vi "WriteToServer.vi"(0 "TCP in":refnum<k5>, 7 "Command":string, 11 "error in":errorcluster, 12 "Timeout(1000ms)":i32=1000) -> (4 "TCP out":refnum<k5>, 6 "ReplyData":T1, 10 "Reply Type":T2, 15 "error out":errorcluster)   [LabVIEW 2020, in "Redis.lvclass"]
uses:
  Redis.lvclass
  ReplyDataTypeEnum.ctl
  ReplyDataType.ctl
  Redis.lvclass/Redis.ctl
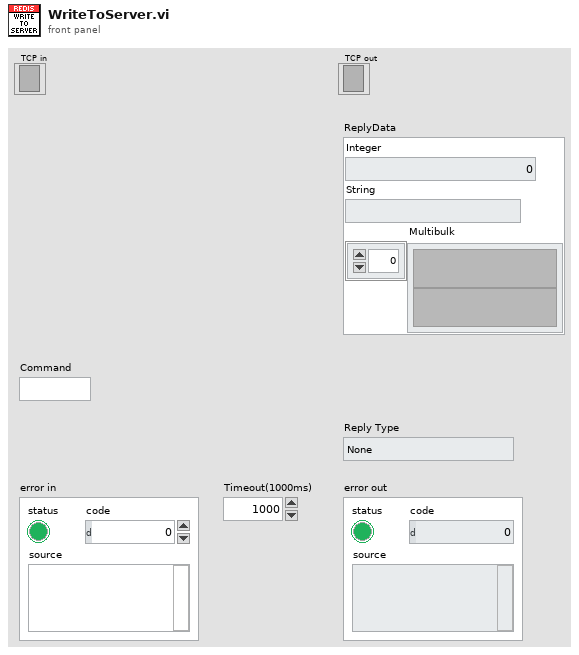
[diagram p1: front panel]
types:
  T1 = typedef "Redis.lvclass/ReplyDataType.ctl" = cluster{"Integer":i64, "String":string, "Multibulk":variant[]}
  T2 = typedef "Redis.lvclass/ReplyDataTypeEnum.ctl" = enum16{"None", "Error", "Status", "Nil", "Integer", "String", "Multibulk"}
  T3 = enum16{"Standard", "Buffered", "CRLF", "Immediate"}
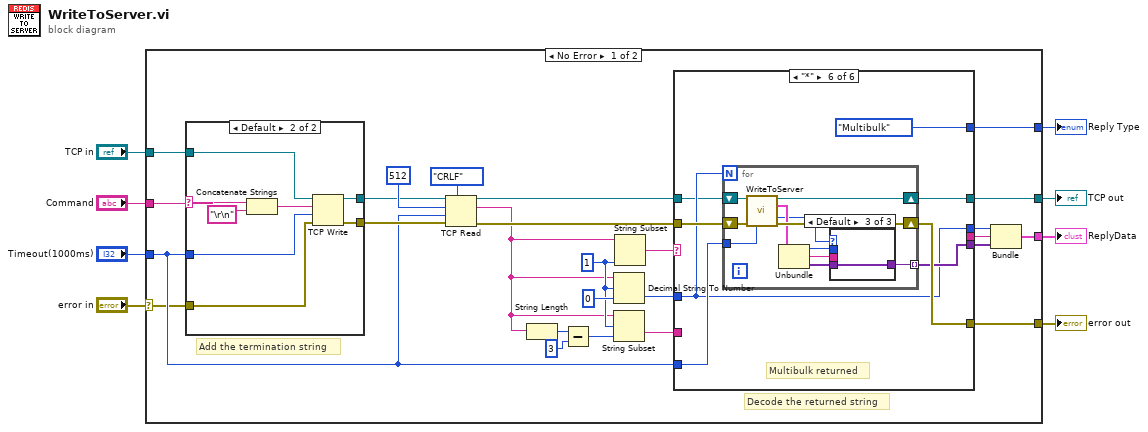
[diagram p0: block diagram]
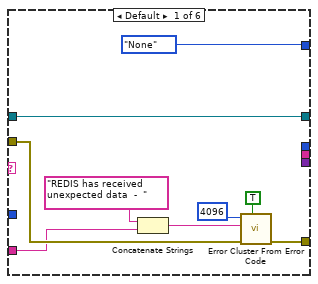
[diagram p3: hidden frame]
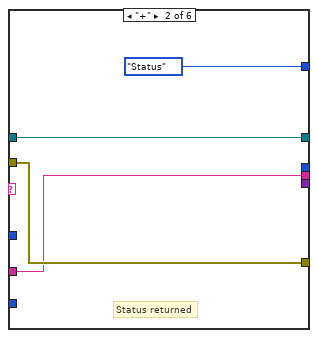
[diagram p4: hidden frame]
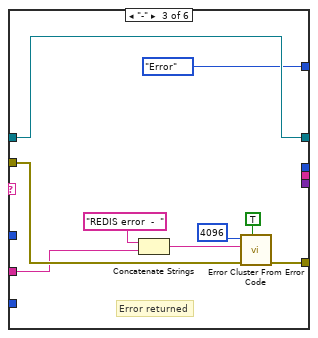
[diagram p5: hidden frame]
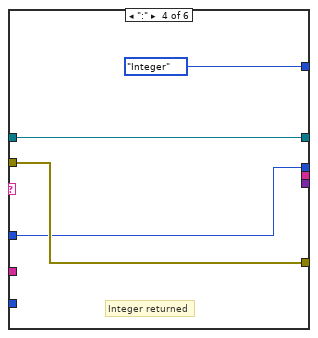
[diagram p6: hidden frame]
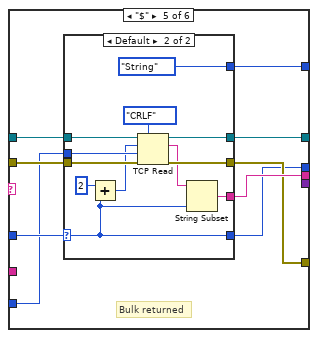
[diagram p7: hidden frame]
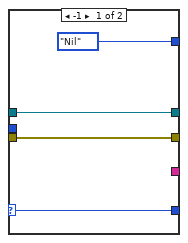
[diagram p8: hidden frame]
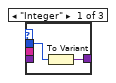
[diagram p9: hidden frame]
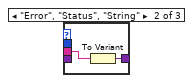
[diagram p10: hidden frame]
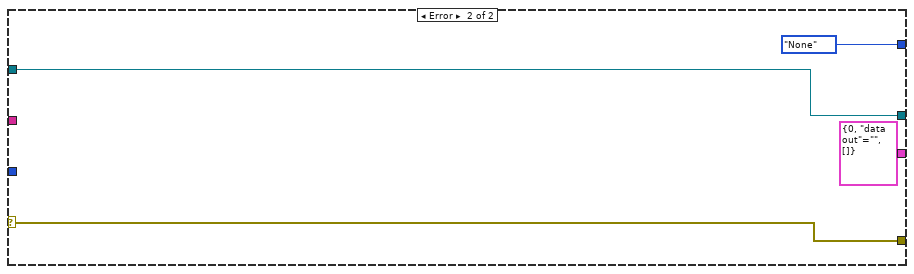
[diagram p11: hidden frame]
diagram:
  n1 = case shown="No Error" "error in" {
    selector: "error in" -> [w9 w122]
    tunnel: [w29 w122] -> w3
    tunnel: [w28 ReplyDataTypeEnum."None" ("Reply Type")] -> w6
    tunnel: "Timeout(1000ms)" -> [w17 _]
    tunnel: "TCP in" -> [w16 w123]
    tunnel: "Command" -> [w15 _]
    tunnel: [w13 cluster{i64, "data out":string, variant[]} {0, "data out"="", []}] -> w1
    tunnel: [w11 w123] -> w7
    frame No Error {
      w24 = 1 ("length (rest)")
      # "Decode the returned string"
      # "Add the termination string"
      n2 = case shown="Default" w15 {
        selector: w15 -> [_ w37]
        tunnel: [w36 w44] -> w12
        tunnel: [w35 w43] -> w18
        tunnel: w9 -> [w35 w42]
        tunnel: w17 -> [_ w41]
        tunnel: w16 -> [w36 w40]
        frame "" {
        }
        frame Default {
          n3 = Concatenate Strings(w37, "\r\n" ("data in")) -> (w39:string)
          n4 = TCP Write(connection ID=w40, data in=w39, error in (no error)=w42, 9:w41) -> (connection ID out=w44:refnum<k5>, error out=w43:errorcluster)  [unwired: 1 out]
        }
      }
      n5 = TCP Read(connection ID=w12, bytes to read=512, error in (no error)=w18, 7:T3."CRLF" ("mode (standard)"), 9:w17) -> (connection ID out=w10:refnum<k5>, data out=w19:string, error out=w30:errorcluster)
      n6 = String Length(string=w19) -> (length=w23:i32)
      n7 = Subtract(x=w23, y=3) -> (x-y=w21:i32)
      n8 = Decimal String To Number(string=w19, offset=w24, default (0L)=i64 0 ("default (0 I32)")) -> (number=w34:i64)  [unwired: 1 out]
      n9 = String Subset(string=w19, offset (0)=w24, length (rest)=w21) -> (substring=w20:string)
      n10 = String Subset(string=w19, length (rest)=w24) -> (substring=w25:string)  [unwired: 1 in]
      n11 = case shown="\"*\"" w25 {
        tunnel: w20 -> [w48 w56 w61 _ _ _]
        tunnel: [_ w56 _ _ w78 _] -> w26
        tunnel: w10 -> [w46 w55 w59 w68 w72 w97]
        tunnel: w34 -> [_ _ _ w69 w79 w99]
        tunnel: [_ _ _ w69 w73 w99] -> w27
        tunnel: [ReplyDataTypeEnum."None" ("Reply Type") ReplyDataTypeEnum."Status" ("Reply Type") ReplyDataTypeEnum."Error" ("Reply Type") ReplyDataTypeEnum."Integer" ("Reply Type") w77 ReplyDataTypeEnum."Multibulk" ("Reply Type")] -> w28
        tunnel: w30 -> [w49 w57 w62 w70 w76 w103]
        tunnel: [w53 w57 w66 w70 w74 w102] -> w29
        tunnel: w17 -> [_ _ _ _ w75 w100]
        tunnel: [_ _ _ _ _ w101] -> w14
        tunnel: [w46 w55 w59 w68 w71 w98] -> w11
        frame Default {
          n12 = Concatenate Strings("REDIS has received unexpected data  -  " ("string"), w48) -> (w51:string)
          n13 = call <vilib>:"Error Cluster From Error Code.vi"("show call chain? (False)"=TRUE, "error in (no error)"=w49, "error message (\"\")"=w51, "error code (0)"=4096) -> ("error out"=w53:errorcluster)  [unwired: 5 in]
        }
        frame "+" {
          # "Status returned"
        }
        frame "-" {
          # "Error returned"
          n14 = Concatenate Strings("REDIS error  -  " ("string"), w61) -> (w64:string)
          n15 = call <vilib>:"Error Cluster From Error Code.vi"("show call chain? (False)"=TRUE, "error in (no error)"=w62, "error message (\"\")"=w64, "error code (0)"=4096) -> ("error out"=w66:errorcluster)  [unwired: 5 in]
        }
        frame ":" {
          # "Integer returned"
        }
        frame "$" {
          # "Bulk returned"
          n16 = case shown="Default" w79 {
            selector: w79 -> [w83 w85]
            tunnel: [_ w87] -> w78
            tunnel: [ReplyDataTypeEnum."Nil" ("Reply Type") ReplyDataTypeEnum."String" ("Reply Type")] -> w77
            tunnel: [w83 w85] -> w73
            tunnel: w76 -> [w82 w94]
            tunnel: w75 -> [_ w93]
            tunnel: [w82 w92] -> w74
            tunnel: w72 -> [w81 w91]
            tunnel: [w81 w86] -> w71
            frame -1 {
            }
            frame Default {
              n17 = Add(x=i64 2, y=w85) -> (x+y=w90:i64)
              n18 = TCP Read(connection ID=w91, bytes to read=w90, error in (no error)=w94, 7:T3."CRLF" ("mode (standard)"), 9:w93) -> (connection ID out=w86:refnum<k5>, data out=w88:string, error out=w92:errorcluster)
              n19 = String Subset(string=w88, length (rest)=w85) -> (substring=w87:string)  [unwired: 1 in]
            }
          }
        }
        frame "*" {
          # "Multibulk returned"
          n20 = for {
            N: w99 -> [_]
            shift-right: [w107] -> w102
            shift-left: w103 -> [w108]
            tunnel: [w114] -> w101 mode=indexing
            tunnel: w100 -> [w104]
            shift-right: [w109] -> w98
            shift-left: w97 -> [w110]
            n21 = call "WriteToServer.vi"("TCP in"=w110, "error in"=w108, "Timeout(1000ms)"=w104) -> ("TCP out"=w109:refnum<k5>, "ReplyData"=w106:T1, "Reply Type"=w105:T2, "error out"=w107:errorcluster)  [unwired: 9 in]
            n22 = Unbundle(w106) -> ("Integer"=w112:i64, "String"=w113:string, "Multibulk"=w111:variant[])
            n23 = case shown="Default" w105 {
              tunnel: w111 -> [_ _ w119]
              tunnel: [w116 w117 w119] -> w114
              tunnel: w112 -> [w115 _ _]
              tunnel: w113 -> [_ w118 _]
              frame "Integer" {
                n24 = To Variant(anything=w115) -> (Variant=w116:variant)
              }
              frame "Error", "Status", "String" {
                n25 = To Variant(anything=w118) -> (Variant=w117:variant)
              }
              frame Default {
              }
            }
          }
        }
      }
      n26 = Bundle(w27, "data out"=w26, w14) -> (w13:cluster{i64, "data out":string, variant[]})  [unwired: 1 in]
    }
    frame Error {
    }
  }
  "TCP out" <- w7
  "Reply Type" <- w6
  "error out" <- w3
  "ReplyData" <- w1
